vi "LimaJapan Fighter.vi"() -> ()   [LabVIEW 2014]
doc: "Simple joystick handling, sensing joystick input in one loop and second handling buttons and som user actions. These loops are independent so you can specify their timing to have different sensitivity.\nName of this VI is just random spelling words from radioamateur communication."
uses:
  <vilib>/Utility/inputDevices.llb/joystickAcquire.vi
  <vilib>/Utility/inputDevices.llb/closeJoystick.vi
  Joystick Fight Simulator.lvlib
panel:
  in  "user input sampling time (ms)":i32=120
  in  "error in":errorcluster
  in  "stop":bool
  out "XY Graph":cluster{i32[], i32[]}(graph)
  out "joystick info":T1(array[cluster])
  out "device name":string
  out "Can't find device":bool
  out "error out":errorcluster
  # "Show joystick movement, limited memory."
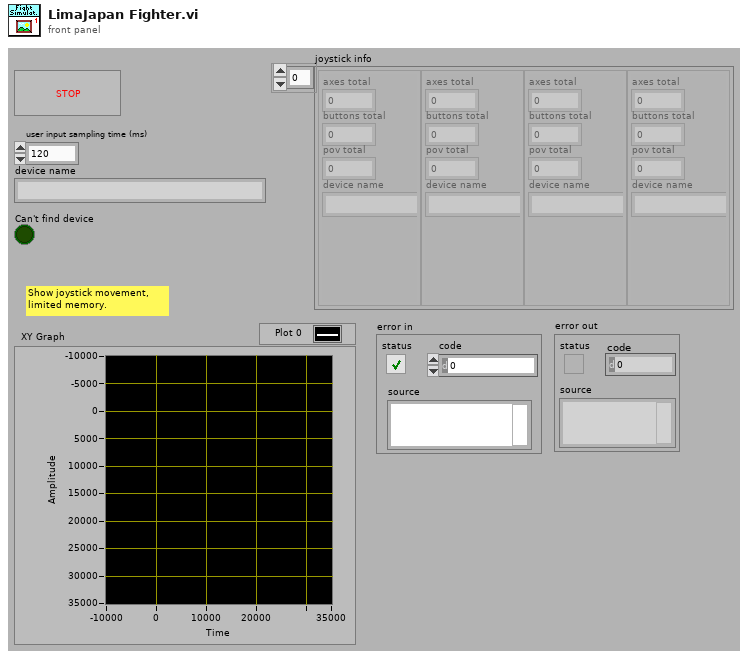
[diagram p1: front panel]
types:
  T1 = cluster{"axes total":u32, "buttons total":u32, "pov total":u32, "device name":string}[]
  T2 = cluster{"X axis":i32, "Y axis":i32, "Z axis":i32, "X axis rotation":i32, "Y axis rotation":i32, "Z axis rotation":i32, "U axis":i32, "V axis":i32}
  T3 = cluster{"button 1":bool, "button 2":bool, "button 3":bool, "button 4":bool, "button 5":bool, "button 6":bool, "button 7":bool, "button 8":bool, "button 9":bool, "button 10":bool, "button 11":bool, "button 12":bool, "button 13":bool, "button 14":bool, "button 15":bool, "button 16":bool, "button 17":bool, "button 18":bool, "button 19":bool, "button 20":bool, "button 21":bool, "button 22":bool, "button 23":bool, "button 24":bool, "button 25":bool, "button 26":bool, "button 27":bool, "button 28":bool, "button 29":bool, "button 30":bool, "button 31":bool, "button 32":bool}
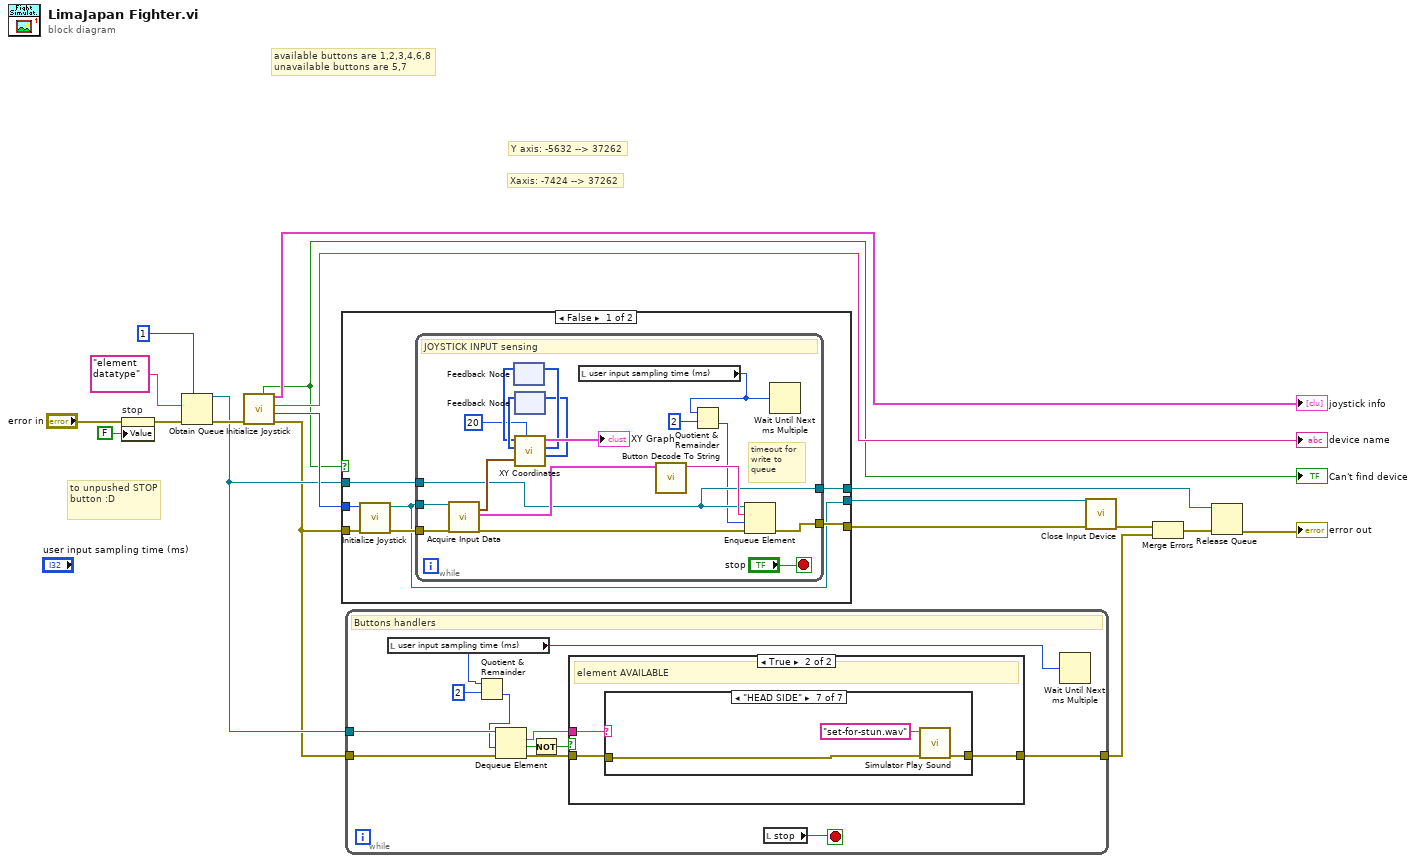
[diagram p0: block diagram]
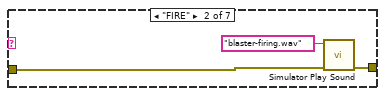
[diagram p4: hidden frame]
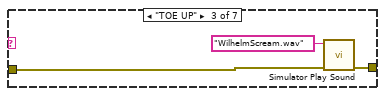
[diagram p5: hidden frame]
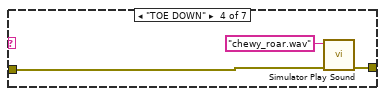
[diagram p6: hidden frame]
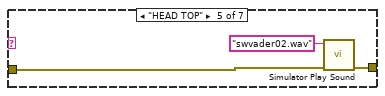
[diagram p7: hidden frame]
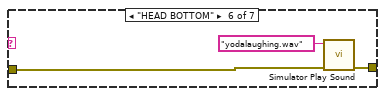
[diagram p8: hidden frame]
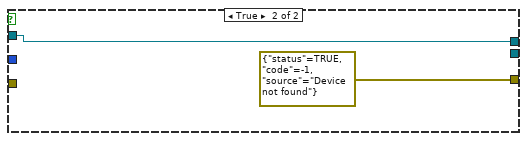
[diagram p9: hidden frame]
diagram:
  # "to unpushed STOP button :D"
  # "Xaxis: -7424 --> 37262"
  # "Y axis: -5632 --> 37262"
  # "available buttons are 1,2,3,4,6,8\nunavailable buttons are 5,7"
  n1 = property on="stop" class="Bool (strict)"(error in="error in", "Value"=FALSE ("stop")) -> (error out=w6:errorcluster)  [unwired: 1 in, 1 out]
  n2 = Obtain Queue(max queue size (-1, unlimited)=1, element data type="element datatype", error in (no error)=w6) -> (queue out=w11:refnum<queue>, error out=w12:errorcluster)  [unwired: 2 in, 1 out]
  n3 = call <vilib>:"Initialize Joystick.vi"("error in (no error)"=w12) -> ("error out"=w10:errorcluster, "input devices count"=w19:i32, "device name"=→"device name":string, "joystick info"=→"joystick info":T1, "Can't find device"=w13:bool)  [unwired: 6 in]
  "Can't find device" <- w13
  n4 = case shown="False" w13 {
    tunnel: w19 -> [w26 _]
    tunnel: [w24 errorcluster {"status"=TRUE, "code"=-1, "source"="Device not found"} ("error out")] -> w18
    tunnel: [w23 _] -> w17
    tunnel: w10 -> [w22 _]
    tunnel: w11 -> [w21 w45]
    tunnel: [w20 w45] -> w2
    frame False {
      n5 = call <vilib>:"Initialize Joystick.vi"("error in (no error)"=w22, "device index"=w26) -> ("error out"=w25:errorcluster, "device ID"=w23:refnum<k1>)  [unwired: 8 in]
      n6 = while {
        tunnel: w25 -> [w44]
        tunnel: w23 -> [w43]
        tunnel: [w34] -> w24
        tunnel: w21 -> [w30]
        tunnel: [w30] -> w20
        stop <- "stop" stop-if-true
        # "timeout for\nwrite to\nqueue"
        # "JOYSTICK INPUT sensing"
        n7 = call-poly <vilib>:"Acquire Input Data.vi"("device ID"=w43, "error in (no error)"=w44) -> ("axis info"=w42:T2, "button info"=w32:T3, "error out"=w33:errorcluster)  [unwired: 13 in, 2 out]
        n8 = feedback #1() -> (w37:i32[])  [unwired: 1 in]
        n9 = feedback #2() -> (w38:i32[])  [unwired: 1 in]
        n10 = call "XY Coordinates.vi"("axis info"=w42, "data history length (samples)"=20, "Y coords"=w38, "X coords"=w37) -> ("Y coords[]"=w39:i32[], "X coords[]"=w40:i32[], "XY Graph"=→"XY Graph":cluster{i32[], i32[]})  [unwired: 5 in]
        n11 = feedback-in #1(w40) -> ()
        n12 = feedback-in #2(w39) -> ()
        n13 = local read "user input sampling time (ms)"() -> (w28:i32)
        n14 = call "Button Decode To String.vi"("button info"=w32) -> ("decoded button string"=w31:string)  [unwired: 10 in]
        n15 = Quotient & Remainder(x=w28, y=2) -> (floor(x/y)=w27:i32)  [unwired: 1 out]
        n16 = Enqueue Element(queue=w30, element=w31, timeout in ms (-1)=w27, error in (no error)=w33) -> (error out=w34:errorcluster)  [unwired: 2 out]
        n17 = Wait Until Next ms Multiple(millisecond multiple=w28) -> ()  [unwired: 1 out]
      }
    }
    frame True {
    }
  }
  n18 = while {
    tunnel: w11 -> [w57]
    tunnel: w10 -> [w56]
    tunnel: [w50] -> w8
    stop <- w55 stop-if-true
    # "Buttons handlers"
    n19 = local read "user input sampling time (ms)"() -> (w48:i32)
    n20 = Quotient & Remainder(x=w48, y=2) -> (floor(x/y)=w47:i32)  [unwired: 1 out]
    n21 = Dequeue Element(queue=w57, timeout in ms (-1)=w47, error in (no error)=w56) -> (element=w51:string, timed out?=w52:bool, error out=w54:errorcluster)  [unwired: 1 out]
    n22 = Not(x=w52) -> (.not. x?=w53:bool)
    n23 = case shown="True" w53 {
      tunnel: w54 -> [w58 w60]
      tunnel: w51 -> [_ w59]
      tunnel: [w58 w61] -> w50
      frame False {
        # "no element in queue"
      }
      frame True {
        # "element AVAILABLE"
        n24 = case shown="\"HEAD SIDE\"" w59 {
          tunnel: w60 -> [w62 w65 w68 w71 w74 w77 w80]
          tunnel: [w62 w64 w67 w70 w73 w76 w79] -> w61
          frame "NO BUTTON", Default {
          }
          frame "FIRE" {
            n25 = call "Simulator Play Sound.vi"("error in (no error)"=w65, "Sound File Path"="blaster-firing.wav") -> ("error out"=w64:errorcluster)  [unwired: 9 in]
          }
          frame "TOE UP" {
            n26 = call "Simulator Play Sound.vi"("error in (no error)"=w68, "Sound File Path"="WilhelmScream.wav") -> ("error out"=w67:errorcluster)  [unwired: 9 in]
          }
          frame "TOE DOWN" {
            n27 = call "Simulator Play Sound.vi"("error in (no error)"=w71, "Sound File Path"="chewy_roar.wav") -> ("error out"=w70:errorcluster)  [unwired: 9 in]
          }
          frame "HEAD TOP" {
            n28 = call "Simulator Play Sound.vi"("error in (no error)"=w74, "Sound File Path"="swvader02.wav") -> ("error out"=w73:errorcluster)  [unwired: 9 in]
          }
          frame "HEAD BOTTOM" {
            n29 = call "Simulator Play Sound.vi"("error in (no error)"=w77, "Sound File Path"="yodalaughing.wav") -> ("error out"=w76:errorcluster)  [unwired: 9 in]
          }
          frame "HEAD SIDE" {
            n30 = call "Simulator Play Sound.vi"("error in (no error)"=w80, "Sound File Path"="set-for-stun.wav") -> ("error out"=w79:errorcluster)  [unwired: 9 in]
          }
        }
      }
    }
    n31 = local read "stop"() -> (w55:bool)
    n32 = Wait Until Next ms Multiple(millisecond multiple=w48) -> ()  [unwired: 1 out]
  }
  n33 = call-poly <vilib>:"Close Input Device.vi"("error in (no error)"=w18, "device ID"=w17) -> ("error out"=w9:errorcluster)  [unwired: 8 in]
  n34 = Merge Errors(w9, w8) -> (w4:errorcluster)
  n35 = Release Queue(queue=w2, error in (no error)=w4) -> (error out=→"error out":errorcluster)  [unwired: 1 in, 2 out]
